vi "Scripting_FindNodeOnDiagram_1.vi"(0 "ViRef(Ignored If Not Wired)":refnum<vi>, 1 "NodeTypesToSearchFor":string[](array[string]), 2 "Diagram(Ignored If Not Wired)":refnum<vi>, 5 "error in (no error)":errorcluster) -> (15 "Nodes":refnum<vi>[](array[refnum]), 19 "error out":errorcluster)   [LabVIEW 2020]
uses:
  <vilib>/Utility/traverseref.llb/TRef TravTarget.ctl
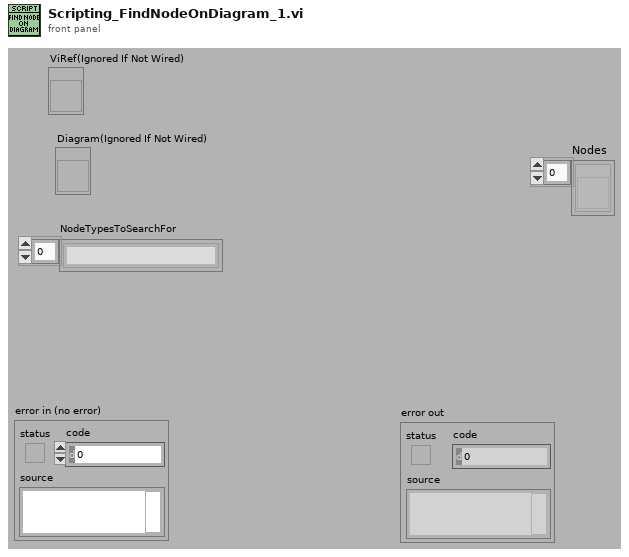
[diagram p1: front panel]
types:
  T1 = typedef "TRef TravTarget.ctl" = enum16{"FP", "BD", "Other"}
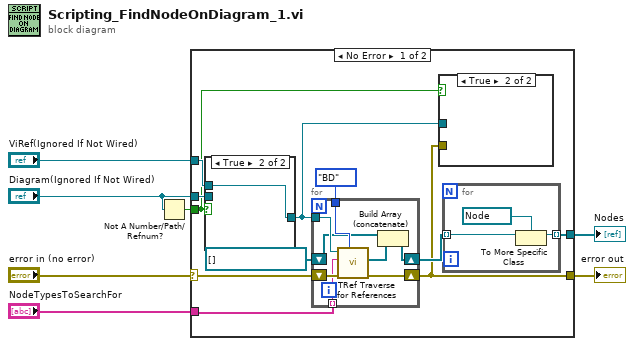
[diagram p0: block diagram]
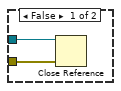
[diagram p2: hidden frame]
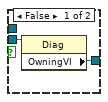
[diagram p3: hidden frame]
diagram:
  n1 = Not A Number/Path/Refnum?(number/path/refnum="Diagram(Ignored If Not Wired)") -> (NaN/Path/Refnum?=w3:bool)
  n2 = case shown="No Error" "error in (no error)" {
    selector: "error in (no error)" -> [w16 w35]
    tunnel: [w9 w35] -> w7
    tunnel: "NodeTypesToSearchFor" -> [w11 _]
    tunnel: "ViRef(Ignored If Not Wired)" -> [w18 _]
    tunnel: w3 -> [w10 _]
    tunnel: "Diagram(Ignored If Not Wired)" -> [w17 _]
    tunnel: [w13 _] -> w1
    frame No Error {
      n3 = case shown="True" w10 {
        tunnel: w18 -> [_ w34]
        tunnel: w17 -> [w33 _]
        tunnel: [w32 w34] -> w8
        frame False {
          n4 = property class="Diag"(reference=w33) -> ("OwningVI"=w32:refnum<vi>)  [unwired: 1 in, 2 out]
        }
        frame True {
        }
      }
      n5 = for {
        tunnel: w8 -> [w28]
        tunnel: TRef_TravTarget."BD" ("Traverse Target") -> [w26]
        shift-right: [w22] -> w14
        shift-left: refnum<vi>[] [] ("References") -> [w24]
        shift-right: [w25] -> w9
        shift-left: w16 -> [w27]
        tunnel: w11 -> [w21] mode=indexing
        n6 = call <vilib>:"TRef Traverse for References.vi"("Traverse Target"=w26, "error in (no error)"=w27, "Class Name"=w21, "VI Refnum"=w28) -> ("error out"=w25:errorcluster, "References"=w23:refnum<vi>[])  [unwired: 4 in, 2 out]
        n7 = Build Array (concatenate)(w24, w23) -> (w22:refnum<vi>[])
      }
      n8 = case shown="True" w10 {
        tunnel: w9 -> [w20 _]
        tunnel: w8 -> [w19 _]
        frame False {
          n9 = Close Reference(reference=w19, error in (no error)=w20) -> ()  [unwired: 1 out]
        }
        frame True {
        }
      }
      n10 = for {
        tunnel: w14 -> [w31] mode=indexing
        tunnel: [w29] -> w13 mode=indexing
        n11 = To More Specific Class(target class=refnum<vi> refnum ("WhileLoop"), reference=w31) -> (specific class reference=w29:refnum<vi>)  [unwired: 1 in, 1 out]
      }
    }
    frame Error {
    }
  }
  "error out" <- w7
  "Nodes" <- w1
